vi "readTelemetryIMSData.vi"(8 "error in (no error)":errorcluster, 10 "Parser":refnum<class "U8ArrayParserAutoIndexing.lvclass">, 11 "M1M3SAL in":refnum<class "M1M3SAL.lvclass">) -> (0 "error out":errorcluster, 2 "EventSummaryState":variant, 3 "M1M3SAL out":refnum<class "M1M3SAL.lvclass">)   [LabVIEW 2016, in "M1M3SupportCommunicator.lvlib" / "M1M3SAL.lvclass"]
uses:
  M1M3SAL.lvclass
  Common_RT_Utilities/U8ArrayParserAutoIndexing/U8ArrayParserAutoIndexing.lvclass
  DataTypes/Topics/TelemetryIMSData.ctl
  DataTypes/Topics/Parts/Timestamp.ctl
  DataTypes/Topics/M1M3SupportTopics.lvlib
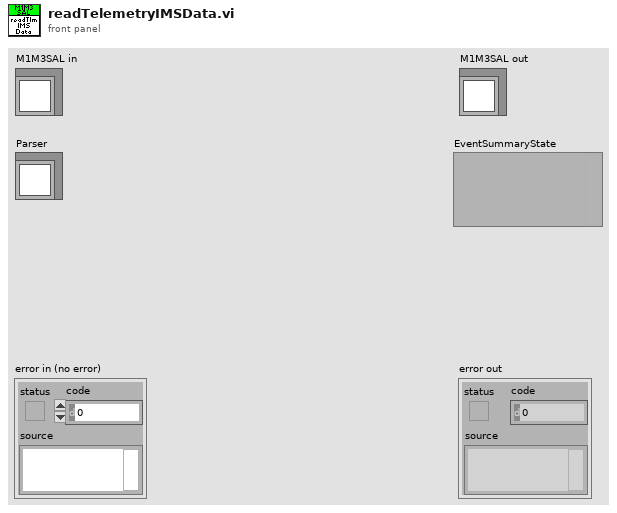
[diagram p1: front panel]
types:
  T1 = typedef "M1M3SupportTopics.lvlib/TelemetryIMSData.ctl" = cluster{"Timestamp":T2, "XPosition":dbl, "YPosition":dbl, "ZPosition":dbl, "XRotation":dbl, "YRotation":dbl, "ZRotation":dbl}
  T2 = typedef "M1M3SupportTopics.lvlib/Timestamp.ctl" = dbl
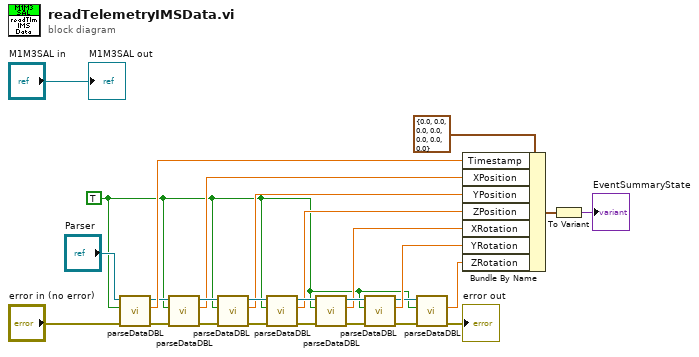
[diagram p0: block diagram]
diagram:
  w1 = TRUE ("OverrideSwapBytes")
  n1 = call "parseDataDBL.vi"("error in (no error)"="error in (no error)", "OverrideSwapBytes"=w1, "U8ArrayParserAutoIndexing in"="Parser") -> ("error out"=w13:errorcluster, "Data"=w22:dbl, "U8ArrayParserAutoIndexing out"=w15:refnum<class "U8ArrayParserAutoIndexing.lvclass">)  [unwired: 6 in]
  n2 = call "parseDataDBL.vi"("error in (no error)"=w13, "OverrideSwapBytes"=w1, "U8ArrayParserAutoIndexing in"=w15) -> ("error out"=w12:errorcluster, "Data"=w11:dbl, "U8ArrayParserAutoIndexing out"=w14:refnum<class "U8ArrayParserAutoIndexing.lvclass">)  [unwired: 6 in]
  n3 = call "parseDataDBL.vi"("error in (no error)"=w12, "OverrideSwapBytes"=w1, "U8ArrayParserAutoIndexing in"=w14) -> ("error out"=w21:errorcluster, "Data"=w10:dbl, "U8ArrayParserAutoIndexing out"=w20:refnum<class "U8ArrayParserAutoIndexing.lvclass">)  [unwired: 6 in]
  n4 = call "parseDataDBL.vi"("error in (no error)"=w21, "OverrideSwapBytes"=w1, "U8ArrayParserAutoIndexing in"=w20) -> ("error out"=w19:errorcluster, "Data"=w9:dbl, "U8ArrayParserAutoIndexing out"=w18:refnum<class "U8ArrayParserAutoIndexing.lvclass">)  [unwired: 6 in]
  n5 = call "parseDataDBL.vi"("error in (no error)"=w19, "OverrideSwapBytes"=w1, "U8ArrayParserAutoIndexing in"=w18) -> ("error out"=w17:errorcluster, "Data"=w8:dbl, "U8ArrayParserAutoIndexing out"=w16:refnum<class "U8ArrayParserAutoIndexing.lvclass">)  [unwired: 6 in]
  n6 = call "parseDataDBL.vi"("error in (no error)"=w17, "OverrideSwapBytes"=w1, "U8ArrayParserAutoIndexing in"=w16) -> ("error out"=w5:errorcluster, "Data"=w7:dbl, "U8ArrayParserAutoIndexing out"=w6:refnum<class "U8ArrayParserAutoIndexing.lvclass">)  [unwired: 6 in]
  n7 = call "parseDataDBL.vi"("error in (no error)"=w5, "OverrideSwapBytes"=w1, "U8ArrayParserAutoIndexing in"=w6) -> ("error out"=→"error out":errorcluster, "Data"=w3:dbl)  [unwired: 6 in, 1 out]
  n8 = Bundle By Name(cluster=T1 {"Timestamp"=0.0, "XPosition"=0.0, "YPosition"=0.0, "ZPosition"=0.0, "XRotation"=0.0, "YRotation"=0.0, "ZRotation"=0.0} ("TelemetryIMSData"), "Timestamp"=w22, "XPosition"=w11, "YPosition"=w10, "ZPosition"=w9, "XRotation"=w8, "YRotation"=w7, "ZRotation"=w3) -> (w26:T1)
  n9 = To Variant(anything=w26) -> (Variant=→"EventSummaryState":variant)
  "M1M3SAL out" <- "M1M3SAL in"
